vi "ENA_recorder.vi"() -> ()   [LabVIEW 2023, in "Recorder.lvlib"]
uses:
  Recorder.lvlib
  lib/CTL/Keysight_VNA.ctl
  lib/Keysight/Keysight.lvlib
panel:
  in  "stop":bool
  in  "Waiting Time(ms)":u32=100
  in  "sParameter":i32=21
  in  "Step_Freq(GHz)":dbl=0.5 format="%#_13g"
  in  "Stop_Freq(GHz)":dbl=31.5
  in  "Start_Freq(GHz)":dbl=26.5
  in  "Polarity":u16(ring) items=["H", "V"]
  in  "TRXmode":u16(ring)=1 items=["Rx"=2, "Tx"=1]
  out "Marker_array":dbl[](array[numeric])
  out "Phase":dbl[][](graph)
  in  "FileName_Note":string
  in  "VISA resource name":refnum<visa-resource-name>="TCPIP0::192.168.100.12::inst0::INSTR"
  out "Return State":bool
  out "output cluster":T1={"address"="192.168.100.111", "remote port or service name"=5025, "timeout ms (60000)"=10000}
  out "Gain":dbl[][](graph)
  out "error out":errorcluster
  # "Setting"
  # "ENA-Recorder"
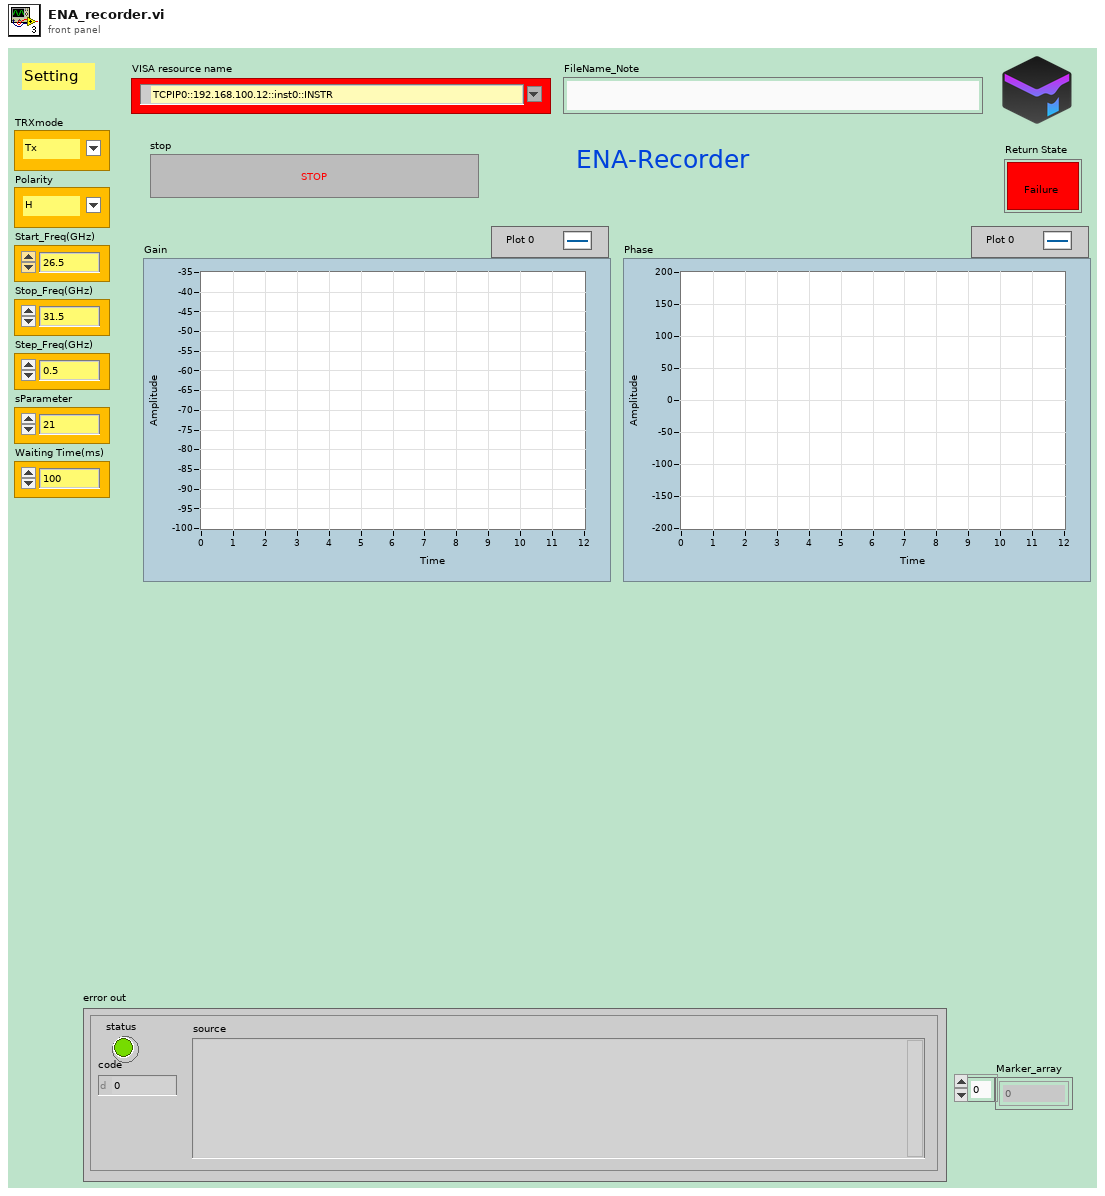
[diagram p1: front panel]
types:
  T1 = cluster{"address":string, "remote port or service name":u16, "timeout ms (60000)":i32}
  T2 = typedef "Keysight_VNA.ctl" = enum16{"Init", "queryMarker", "setSweepPoint", "setMarkerFreq", "setMeasureFormat", "setFreqStartStop", "setMarkerOnOFF", "setMarkerFormat_LOGP", "setMeasPAR_S", "setTriggerSingle", "Trigger_Save_SnP", "Trigger_Single", "Close"}
  T3 = cluster{"setSweepPoint":i32, "Meas":i32, "Mark":i32, "Freq_GHz":dbl, "Start_Freq(GHz)":dbl, "Stop_Freq(GHz)":dbl, "sParameter":i32}
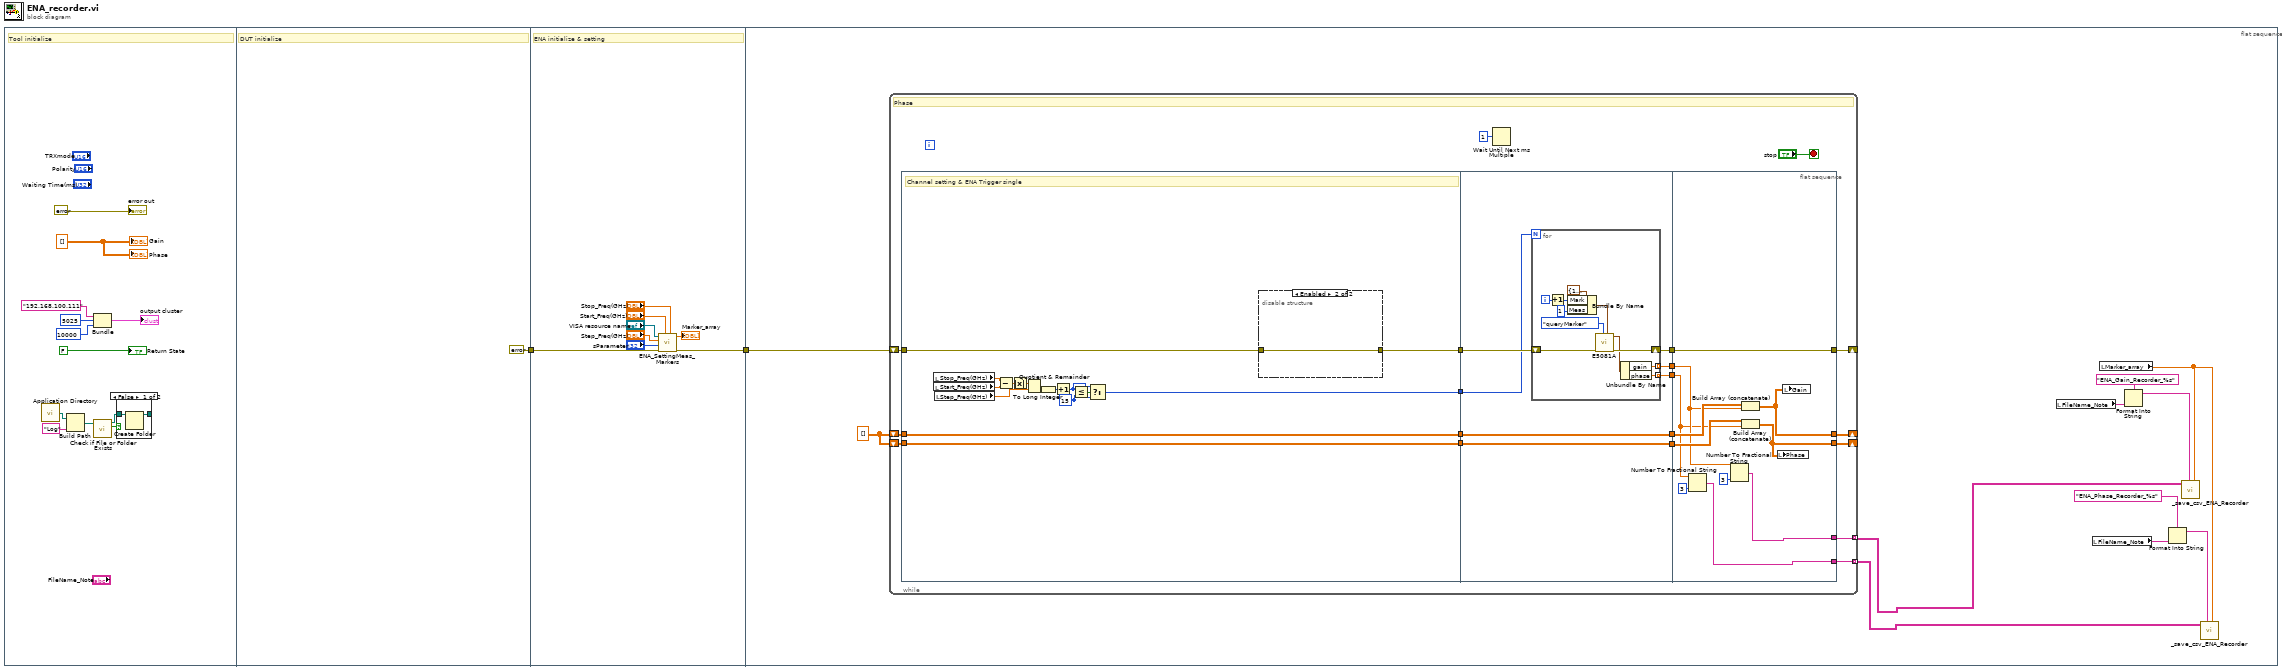
[diagram p0: block diagram]
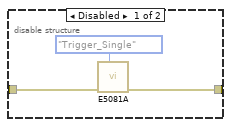
[diagram p3: hidden frame]
diagram:
  n1 = flat-sequence {
    tunnel: [errorcluster {"status"=FALSE, "code"=0, "source"=""} ("error out")] -> w2
    tunnel: w2 -> [w20]
    tunnel: [w21] -> w1
    tunnel: w1 -> [w37]
    frame #0 {
      w3 = dbl[][] []
      # "Tool initialize"
      n2 = call <vilib>:"Application Directory.vi"() -> ("Application Directory"=w7:path)
      n3 = Build Path(base path=w7, name or relative path="Log") -> (appended path=w4:path)
      n4 = Bundle("address"="192.168.100.111", "remote port or service name"=u16 5025, "timeout ms (60000)"=10000) -> (→"output cluster":T1)  [unwired: 1 in]
      n5 = call <vilib>:"Check if File or Folder Exists.vi"("path"=w4) -> ("file or folder exists?"=w6:bool, "dup path"=w5:path)  [unwired: 8 in, 1 out]
      n6 = case shown="False" w6 {
        tunnel: w5 -> [w16 w17]
        tunnel: [w15 w17] -> _
        frame False {
          n7 = Create Folder(path (use dialog)=w16) -> (created path=w15:path)  [unwired: 2 in, 2 out]
        }
        frame True {
        }
      }
      "error out" <- errorcluster {"status"=FALSE, "code"=0, "source"=""} ("error out")
      "Return State" <- FALSE ("OK?")
      "Gain" <- w3
      "Phase" <- w3
    }
    frame #1 {
      # "DUT initialize"
    }
    frame #2 {
      # "ENA initialize & setting"
      n8 = call "ENA_SettingMeas_Markers.vi"("Stop_Freq(GHz)"="Stop_Freq(GHz)", "Start_Freq(GHz)"="Start_Freq(GHz)", "error in"=w20, "sParameter"="sParameter", "Step_Freq(GHz)"="Step_Freq(GHz)", "VISA IN"="VISA resource name") -> ("error out"=w21:errorcluster, "Marker_array"=→"Marker_array":dbl[])  [unwired: 4 in]
    }
    frame #3 {
      w32 = dbl[][] []
      n9 = while {
        shift-right: [w52] -> _
        shift-left: w37 -> [w56]
        tunnel: [w49] -> w31 mode=indexing
        tunnel: [w48] -> w30 mode=indexing
        shift-right: [w41] -> _
        shift-left: w32 -> [w45]
        shift-right: [w40] -> _
        shift-left: w32 -> [w42]
        stop <- "stop" stop-if-true
        # "Phase"
        n10 = flat-sequence {
          tunnel: w56 -> [w57]
          tunnel: [w58] -> w55
          tunnel: [w61] -> w54
          tunnel: [w60] -> w46
          tunnel: w45 -> [w60]
          tunnel: [w59] -> w43
          tunnel: w42 -> [w59]
          tunnel: w55 -> [w81]
          tunnel: w54 -> [w80]
          tunnel: [w82] -> w53
          tunnel: [w79] -> w51
          tunnel: [w78] -> w50
          tunnel: [w77] -> w47
          tunnel: w46 -> [w77]
          tunnel: [w76] -> w44
          tunnel: w43 -> [w76]
          tunnel: [w96] -> w52
          tunnel: w53 -> [w96]
          tunnel: w51 -> [w100]
          tunnel: w50 -> [w99]
          tunnel: [w95] -> w49
          tunnel: [w94] -> w48
          tunnel: w47 -> [w102]
          tunnel: w44 -> [w101]
          tunnel: [w98] -> w41
          tunnel: [w97] -> w40
          frame #0 {
            w71 = 15 ("y")
            # "Channel setting & ENA Trigger single"
            n11 = local read "Stop_Freq(GHz)"() -> (w64:dbl)
            n12 = local read "Start_Freq(GHz)"() -> (w63:dbl)
            n13 = local read "Step_Freq(GHz)"() -> (w62:dbl)
            n14 = Subtract(x=w64, y=w63) -> (x-y=w70:dbl)
            n15 = Absolute Value(x=w70) -> (abs(x)=w69:dbl)
            n16 = Quotient & Remainder(x=w69, y=w62) -> (floor(x/y)=w68:dbl)  [unwired: 1 out]
            n17 = To Long Integer(number=w68) -> (32bit integer=w67:i32)
            n18 = Increment(x=w67) -> (x+1=w65:i32)
            n19 = Less Or Equal?(x=w65, y=w71) -> (x <= y?=w66:bool)
            n20 = Select(t=w65, s=w66, f=w71) -> (s? t:f=w61:i32)
            n21 = disable-structure shown="Enabled" {
              disable-tunnel: [w73 w75] -> w58
              disable-tunnel: w57 -> [w72 w75]
              frame Disabled {
                n22 = call "E5081A.vi"("Function_VNA"=Keysight_VNA."Trigger_Single", "error in"=w72) -> ("error out"=w73:errorcluster)  [unwired: 8 in, 1 out]
              }
              frame Enabled {
              }
            }
          }
          frame #1 {
            n23 = for {
              N: w80 -> [_]
              shift-right: [w92] -> w82
              shift-left: w81 -> [w93]
              tunnel: [w84] -> w79 mode=indexing
              tunnel: [w83] -> w78 mode=indexing
              i -> [w89]
              n24 = Increment(x=w89) -> (x+1=w87:i32)
              n25 = Bundle By Name(cluster=T3 {"setSweepPoint"=11, "Meas"=1, "Mark"=0, "Freq_GHz"=0.0, "Start_Freq(GHz)"=0.0, "Stop_Freq(GHz)"=0.0, "sParameter"=1} ("Input"), "Mark"=w87, "Meas"=1) -> (w86:T3)
              n26 = call "E5081A.vi"("Input"=w86, "Function_VNA"=Keysight_VNA."queryMarker", "error in"=w93) -> ("error out"=w92:errorcluster, "queryMarker"=w85:cluster{"gain":dbl, "phase":dbl})  [unwired: 7 in]
              n27 = Unbundle By Name(w85) -> ("gain"=w84:dbl, "phase"=w83:dbl)
            }
          }
          frame #2 {
            n28 = Number To Fractional String(number=w99, precision (6)=i16 3) -> (F-format string=w94:string[])  [unwired: 2 in]
            n29 = Number To Fractional String(number=w100, precision (6)=i16 3) -> (F-format string=w95:string[])  [unwired: 2 in]
            n30 = Build Array (concatenate)(w101, w99) -> (w97:dbl[][])
            n31 = Build Array (concatenate)(w102, w100) -> (w98:dbl[][])
            n32 = local write "Phase"(w97) -> ()
            n33 = local write "Gain"(w98) -> ()
          }
        }
        n34 = Wait Until Next ms Multiple(millisecond multiple=u32 1) -> ()  [unwired: 1 out]
      }
      n35 = local read "FileName_Note"() -> (w29:string)
      n36 = local read "FileName_Note"() -> (w27:string)
      n37 = local read "Marker_array"() -> (w36:dbl[])
      n38 = Format Into String(format string="ENA_Gain_Recorder_%s" ("NoteName"), w29) -> (resulting string=w34:string)  [unwired: 2 in, 1 out]
      n39 = Format Into String(format string="ENA_Phase_Recorder_%s" ("NoteName"), w27) -> (resulting string=w33:string)  [unwired: 2 in, 1 out]
      n40 = call "_save_csv_ENA_Recorder.vi"("Marker_array"=w36, "NoteName"=w34, "array in"=w31) -> ()  [unwired: 8 in, 1 out]
      n41 = call "_save_csv_ENA_Recorder.vi"("Marker_array"=w36, "NoteName"=w33, "array in"=w30) -> ()  [unwired: 8 in, 1 out]
    }
  }
